vi "Telemetry Logging Loop.vi"(6 "Log Folder":path, 8 "Log Status Ind":refnum<vi>, 9 "Log File Ind":refnum<vi>, 10 "Log Size Ind":refnum<vi>, 11 "Queue in":refnum<queue>) -> ()   [LabVIEW 2015]
uses:
  Telemetry Packet Type.ctl
  Thermocouple Data.ctl
  Sensors/Transducer Calibration Display.ctl
  Sensors/Sensor Enum.ctl
  Logging/Logger State.ctl
  Logging/Logger Command.ctl
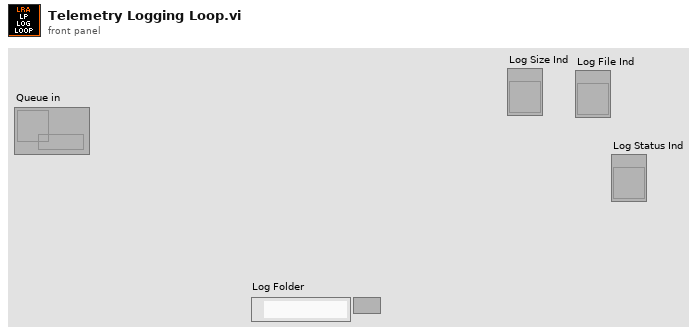
[diagram p1: front panel]
types:
  T1 = typedef "Logger Command.ctl" = enum16{"Init", "Start", "Stop"}
  T2 = typedef "Logger State.ctl" = enum16{"Stopped", "Running"}
  T3 = enum16{"open", "replace", "create", "open or create", "replace or create", "replace or create with confirmation"}
  T4 = typedef "Telemetry Packet Type.ctl" = cluster{"Timestamp\n":u32, "Transducer Value":u16[], "Main Loop Rate":u32, "Solenoid State":bool[], "Output Enabled":bool, "Solenoids Powered":bool, "TC Data":T5[], "TD Rate":u32, "TD Execution Time":u32, "TC Rate":u32, "TC Execution Time":u32, "Decoded Sensor Data":T6[]}
  T5 = typedef "Thermocouple Data.ctl" = cluster{"TC Temp":dbl, "Internal Temp":dbl, "Fault":bool, "Short to VCC":bool, "Short to GND":bool, "Open Circuit":bool}
  T6 = typedef "Transducer Calibration Display.ctl" = cluster{"Value":dbl, "Raw":dbl, "Scaled":dbl, "Sensor Name":T7, "Port":u32}
  T7 = typedef "Sensor Enum.ctl" = enum16{"FPD-1", "FPD-2", "FPD-3", "OPD-1", "OPD-2", "OPD-3", "AP-1", "VBAT", "VCOMP", "ICOMP", "TD10"}
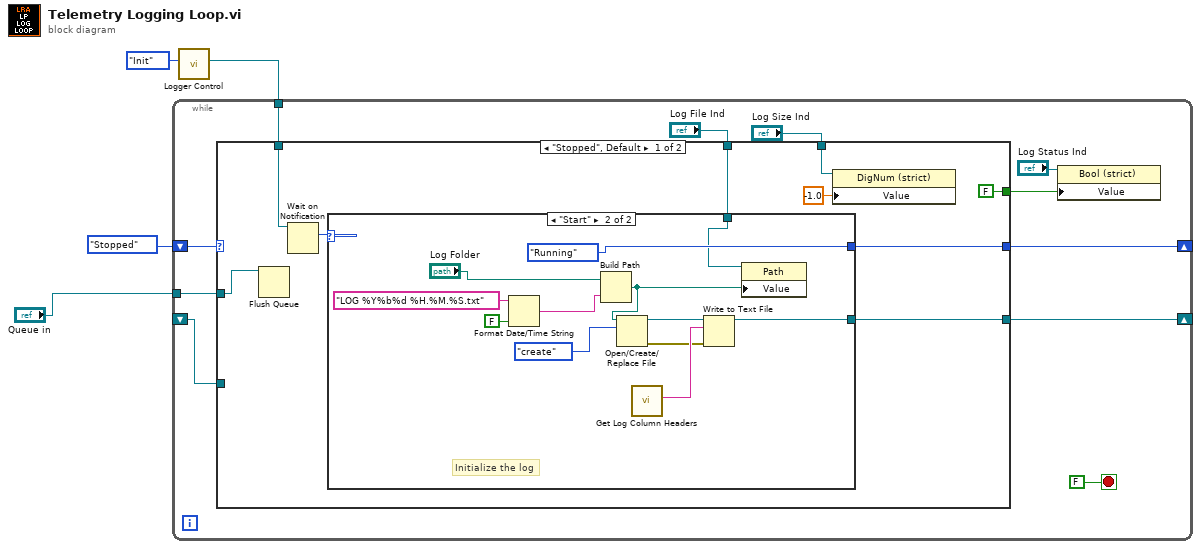
[diagram p0: block diagram]
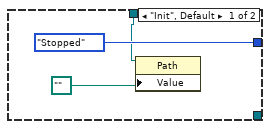
[diagram p2: hidden frame]
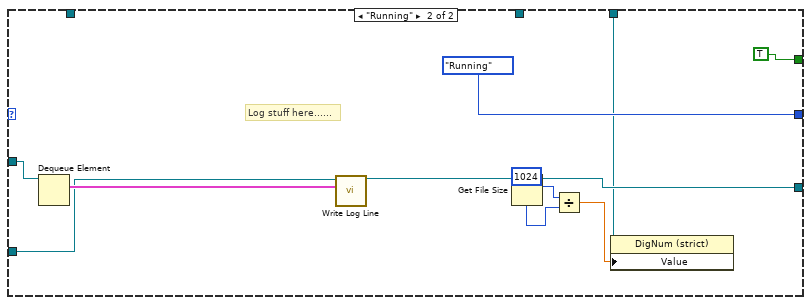
[diagram p3: hidden frame]
diagram:
  n1 = call "Logger Control.vi"("Command"=Logger_Command."Init") -> ("notifier out"=w2:refnum<notifier>)  [unwired: 10 in]
  n2 = while {
    shift-right: [w11] -> _
    shift-left: Logger_State."Stopped" -> [w14]
    tunnel: w2 -> [w13]
    tunnel: "Queue in" -> [w12]
    shift-right: [w10] -> _
    shift-left: _ -> [w9]
    stop <- FALSE stop-if-true
    n3 = case shown="\"Stopped\", Default" w14 {
      tunnel: w13 -> [w24 _]
      tunnel: w12 -> [w21 w50]
      tunnel: [w22 Logger_State."Running"] -> w11
      tunnel: [w20 w45] -> w10
      tunnel: w9 -> [_ w47]
      tunnel: "Log Size Ind" -> [w19 w41]
      tunnel: [FALSE TRUE] -> w6
      tunnel: "Log File Ind" -> [w16 _]
      frame "Stopped", Default {
        n4 = Flush Queue(queue=w21) -> ()  [unwired: 1 in, 3 out]
        n5 = Wait on Notification(notifier=w24) -> (notification=w23:T1)  [unwired: 3 in, 3 out]
        n6 = case shown="\"Start\"" w23 {
          tunnel: [Logger_State."Stopped" Logger_State."Running"] -> w22
          tunnel: [_ w34] -> w20
          tunnel: w16 -> [w26 w31]
          frame "Init", Default {
            n7 = property class="Path"(reference=w26, "Value"=path "") -> ()  [unwired: 1 in, 2 out]
          }
          frame "Start" {
            # "Initialize the log"
            n8 = Format Date/Time String(time format string (%c)="LOG %Y%b%d %H.%M.%S.txt", UTC format=FALSE) -> (date/time string=w28:string)  [unwired: 1 in]
            n9 = Build Path(base path="Log Folder", name or relative path=w28) -> (appended path=w29:path)
            n10 = Open/Create/Replace File(file path (use dialog)=w29, operation (0:open)=T3."create") -> (refnum out=w35:refnum<file>, error out=w32:errorcluster)  [unwired: 4 in, 1 out]
            n11 = call "Get Log Column Headers.vi"() -> ("Headers String"=w33:string)  [unwired: 11 in]
            n12 = Write to Text File(file (use dialog)=w35, text=w33, error in=w32) -> (refnum out=w34:refnum<file>)  [unwired: 1 in, 2 out]
            n13 = property class="Path"(reference=w31, "Value"=w29) -> ()  [unwired: 1 in, 2 out]
          }
        }
        n14 = property class="DigNum (strict)"(reference=w19, "Value"=-1.0) -> ()  [unwired: 1 in, 2 out]
      }
      frame "Running" {
        # "Log stuff here......"
        n15 = Dequeue Element(queue=w50) -> (element=w48:T4)  [unwired: 2 in, 3 out]
        n16 = call "Write Log Line.vi"("Cluster"=w48, "Byte Stream File in"=w47) -> ("Byte Stream File out"=w46:refnum<file>)  [unwired: 9 in]
        n17 = Get File Size(file=w46) -> (refnum out=w45:refnum<file>, size (in bytes)=w44:i64)  [unwired: 1 in, 1 out]
        n18 = Divide(x=w44, y=i64 1024) -> (x/y=w42:dbl)
        n19 = property class="DigNum (strict)"(reference=w41, "Value"=w42) -> ()  [unwired: 1 in, 2 out]
      }
    }
    n20 = property class="Bool (strict)"(reference="Log Status Ind", "Value"=w6) -> ()  [unwired: 1 in, 2 out]
  }
